vi "Set Section.vi"(8 "error in":errorcluster, 9 "Section Definition":T1, 10 "section":string, 11 "key lookup":variant) -> (0 "error out":errorcluster, 3 "key lookup out":variant)   [LabVIEW 2012, in "configlib.lvlib"]
uses:
  configlib.lvlib
  Section Definition.ctl
  File Section.ctl
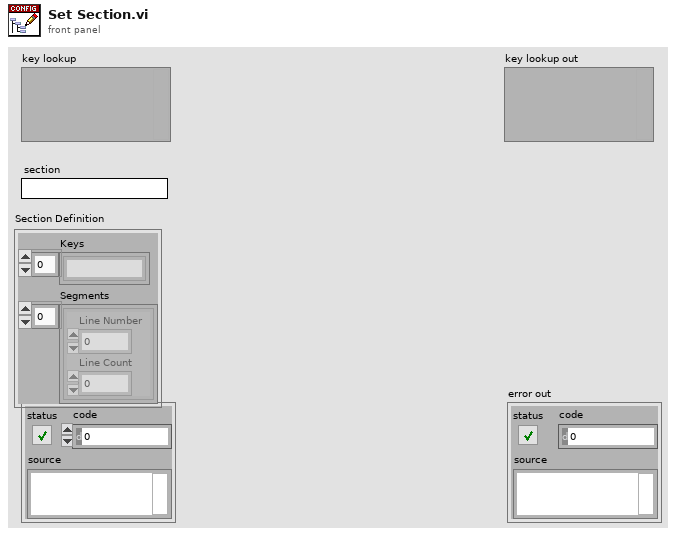
[diagram p1: front panel]
types:
  T1 = typedef "configlib.lvlib/Section Definition.ctl" = cluster{"Keys":string[], "Segments":T2[]}
  T2 = typedef "configlib.lvlib/File Section.ctl" = cluster{"Line Number":i32, "Line Count":i32}
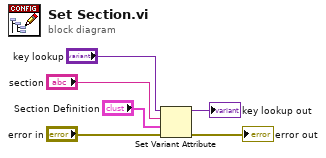
[diagram p0: block diagram]
diagram:
  n1 = Set Variant Attribute(Variant="key lookup", name="section", value="Section Definition", error in="error in") -> (Variant out=→"key lookup out":variant, error out=→"error out":errorcluster)  [unwired: 1 out]
